vi "Set_Get_Path_Info_File.vi"(10 "Add Info File Path (False)":bool, 11 "Info File Path":path) -> (2 "Info File Path Out":path, 3 "Info Path File Out":string)   [LabVIEW 2018]
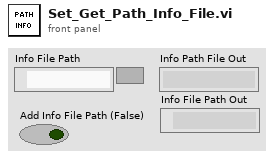
[diagram p1: front panel]
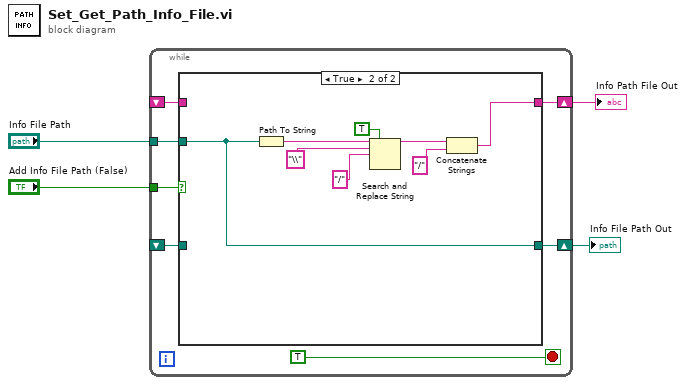
[diagram p0: block diagram]
diagram:
  n1 = while {
    tunnel: "Add Info File Path (False)" -> [w10]
    shift-right: [w9] -> w2
    shift-left: _ -> [w7]
    tunnel: "Info File Path" -> [w8]
    shift-right: [w6] -> w1
    shift-left: _ -> [w5]
    stop <- TRUE stop-if-true
    n2 = case shown="True" w10 {
      tunnel: [w13 w15] -> w9
      tunnel: w8 -> [_ w14]
      tunnel: w7 -> [w13 _]
      tunnel: [w12 w14] -> w6
      tunnel: w5 -> [w12 _]
      frame False {
      }
      frame True {
        n3 = Path To String(path=w14) -> (string=w20:string)
        n4 = Search and Replace String(replace all?=TRUE ("replace all? (F)"), input string=w20, search string="\\", replace string="/" ("replace string (\"\")")) -> (result string=w21:string)  [unwired: 4 in, 3 out]
        n5 = Concatenate Strings(w21, "/" ("string")) -> (w15:string)
      }
    }
  }
  "Info Path File Out" <- w2
  "Info File Path Out" <- w1
